vi "CreateReplace Link.vi"(4 "Replace Existing?":bool=TRUE, 5 "Link Type":T2 items=["H5G_LINK_ERROR"=-1, "H5G_LINK_HARD"=0, "H5G_LINK_SOFT"=1], 6 "HDF5 New Loc (same)":T1, 7 "error in (no error)":errorcluster, 8 "New Name":string, 9 "Current Name":string, 10 "HDF5 Ref":T1) -> (0 "error out":errorcluster, 3 "HDF5 Ref out":T1)   [LabVIEW 2017]
doc: "Creates or replaces a hard or soft link"
uses:
  <vilib>/UPVI/lvhdf5/library.llb/HDF5 Ref.ctl
  <vilib>/UPVI/lvhdf5/group.llb/H5G_link_t.ctl
  <vilib>/UPVI/lvhdf5/identifier.llb/H5Iget_type.vi
panel:
  # "LVHDF5 Toolkit\nCopyright (c) 2005-2013 by Jason D. Sommerville\nCopyright (c) 2014 by UPVI, LLC.\n\nThis use and distribution of this file is governed by the terms found in \nLICENSE.txt distributed with this toolkit and installed at\n <user.lib>\\_lvhdf5\\LICENSE.txt"
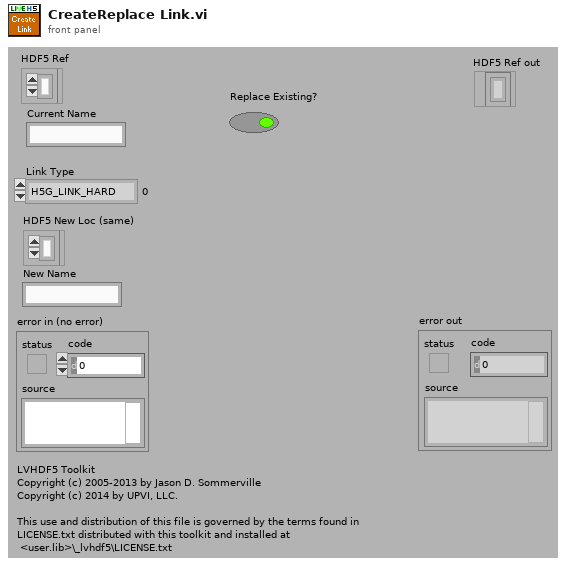
[diagram p1: front panel]
types:
  T1 = typedef "HDF5 Ref.ctl" = refnum<k1>
  T2 = typedef "H5G_link_t.ctl" = i32
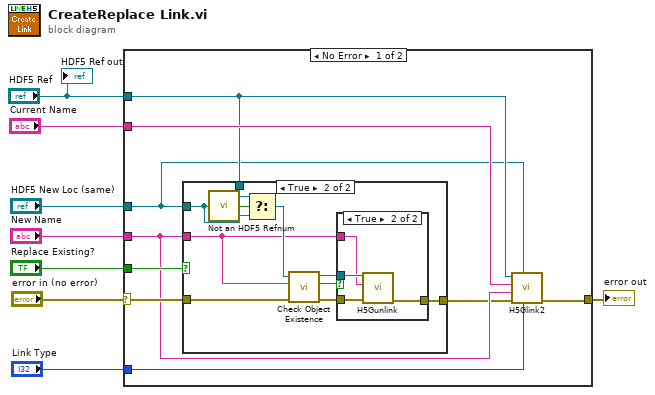
[diagram p0: block diagram]
diagram:
  n1 = case shown="No Error" "error in (no error)" {
    selector: "error in (no error)" -> [w16 w34]
    tunnel: [w9 w34] -> w7
    tunnel: "HDF5 Ref" -> [w11 _]
    tunnel: "Current Name" -> [w12 _]
    tunnel: "New Name" -> [w14 _]
    tunnel: "HDF5 New Loc (same)" -> [w10 _]
    tunnel: "Replace Existing?" -> [w17 _]
    tunnel: "Link Type" -> [w15 _]
    frame No Error {
      n2 = case shown="True" w17 {
        tunnel: w16 -> [w18 w28]
        tunnel: w14 -> [_ w21]
        tunnel: w10 -> [_ w26]
        tunnel: [w18 w20] -> w13
        tunnel: w11 -> [_ w19]
        frame False {
        }
        frame True {
          n3 = call <vilib>:"Not an HDF5 Refnum.vi"("HDF5 Ref"=w26) -> ("Not an HDF5 Refnum"=w27:bool)
          n4 = Select(t=w19, s=w27, f=w26) -> (s? t:f=w25:T1)
          n5 = call <vilib>:"Check Object Existence.vi"("error in (no error)"=w28, "name"=w21, "HDF5 Ref"=w25) -> ("error out"=w24:errorcluster, "Exists"=w23:bool, "HDF5 Ref out"=w22:T1)  [unwired: 4 in]
          n6 = case shown="True" w23 {
            tunnel: w24 -> [w29 w33]
            tunnel: w22 -> [_ w32]
            tunnel: w21 -> [_ w31]
            tunnel: [w29 w30] -> w20
            frame False {
            }
            frame True {
              n7 = call <vilib>:"H5Gunlink.vi"("error in (no error)"=w33, "Name"=w31, "HDF5 Ref"=w32) -> ("error out"=w30:errorcluster)  [unwired: 5 in, 1 out]
            }
          }
        }
      }
      n8 = call <vilib>:"H5Glink2.vi"("Link Type"=w15, "HDF5 New Loc (same)"=w10, "error in (no error)"=w13, "New Name"=w14, "Current Name"=w12, "HDF5 Ref"=w11) -> ("error out"=w9:errorcluster)  [unwired: 4 in, 1 out]
    }
    frame Error {
    }
  }
  "error out" <- w7
  "HDF5 Ref out" <- "HDF5 Ref"
